vi "SwerveDrive.vi"(0 "x":dbl, 1 "offset":dbl, 2 "Wheel":T1(ring)=enum."FrontLeft", 3 "PWM Counters":cluster{"High":dbl, "Low":dbl}, 5 "y":dbl, 9 "z":dbl, 11 "theta (radians)":dbl, 12 "Enabled":bool=TRUE) -> (4 "twist motor power":dbl, 6 "drive motor power":dbl, 10 "aligned":bool, 13 "angle (radians)":dbl, 14 "Angle Error":dbl, 15 "reversed?":bool)   [LabVIEW 2013]
uses:
  <vilib>/addons/control/pid/pid.llb/PID Advanced (DBL).vi
  <vilib>/addons/control/pid/NI_PID_pid.lvlib
panel:
  in  "PID gains":T2={"proportional gain (Kc)"=0.3, "integral time (Ti, min)"=0.01, "derivative time (Td, min)"=0.0} {"derivative time (Td, min)" format="%.3f"; "integral time (Ti, min)" format="%.3f"; "proportional gain (Kc)" format="%.3f"}
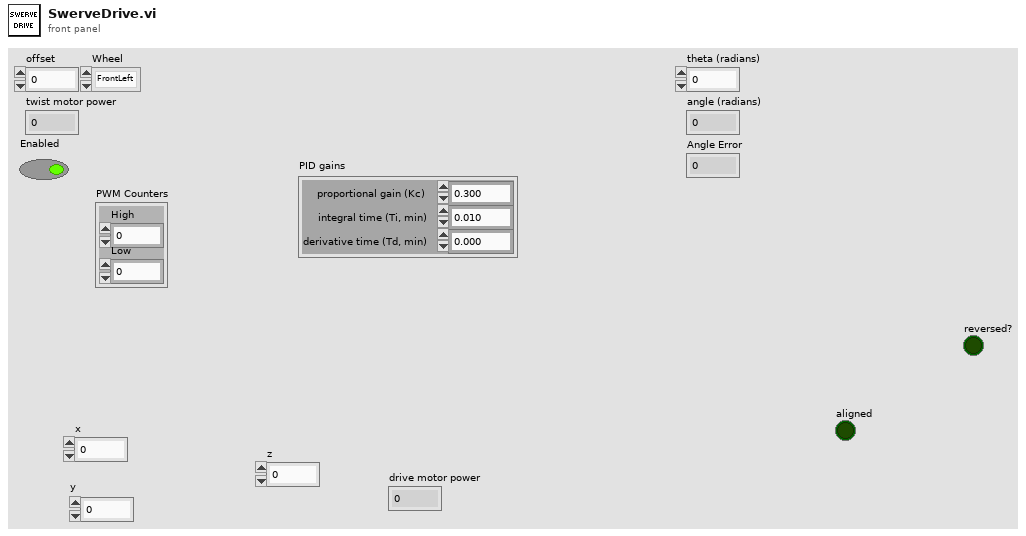
[diagram p1: front panel]
types:
  T1 = enum16{"FrontRight", "FrontLeft", "RearRight", "RearLeft"}
  T2 = cluster{"proportional gain (Kc)":dbl, "integral time (Ti, min)":dbl, "derivative time (Td, min)":dbl}
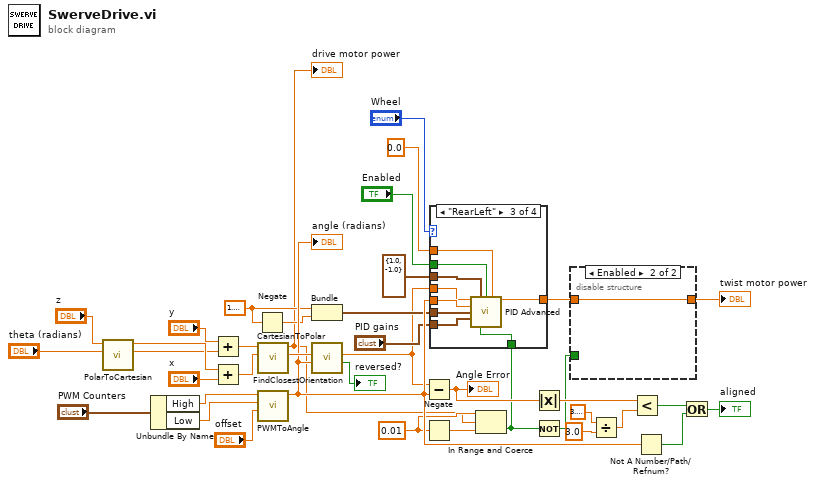
[diagram p0: block diagram]
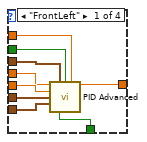
[diagram p2: hidden frame]
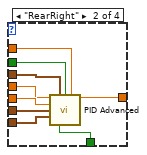
[diagram p3: hidden frame]
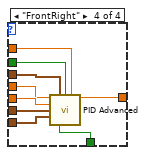
[diagram p4: hidden frame]
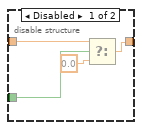
[diagram p5: hidden frame]
diagram:
  w6 = 0.01 ("x")
  w14 = 1.5707963267948966
  n1 = call "PolarToCartesian.vi"("theta (radians)"="theta (radians)", "r"="z") -> ("y"=w35:dbl, "x"=w37:dbl)  [unwired: 8 in]
  n2 = Unbundle By Name("PWM Counters") -> ("High"=w20:dbl, "Low"=w19:dbl)
  n3 = Add(x="y", y=w35) -> (x+y=w29:dbl)
  n4 = Add(x=w37, y="x") -> (x+y=w28:dbl)
  n5 = Negate(x=w14) -> (-x=w13:dbl)
  n6 = call "CartesianToPolar.vi"("y"=w28, "x"=w29) -> ("theta (radians)"=w25:dbl, "r"=w5:dbl)  [unwired: 8 in]
  "drive motor power" <- w5
  n7 = call "PWMToAngle.vi"("official"="offset", "low"=w19, "high"=w20) -> ("angle (radians)"=w16:dbl)  [unwired: 8 in]
  "angle (radians)" <- w16
  n8 = Bundle(w14, w13) -> (w15:cluster{dbl, dbl})  [unwired: 1 in]
  n9 = call "FindClosestOrientation.vi"("current angle (radians)"=w16, "desired angle (radians)"=w25) -> ("reversed?"=→"reversed?":bool, "closest angle (radians)"=w3:dbl)  [unwired: 8 in]
  n10 = Subtract(x=w3, y=w16) -> (x-y=w30:dbl)
  "Angle Error" <- w30
  n11 = Negate(x=w6) -> (-x=w7:dbl)
  n12 = In Range and Coerce(upper limit=w6, x=w5, lower limit=w7) -> (In Range?=w1:bool)  [unwired: 1 out]
  n13 = case shown="\"RearLeft\"" "Wheel" {
    tunnel: w16 -> [w48 w57 w66 w75]
    tunnel: w15 -> [w47 w56 w65 w74]
    tunnel: cluster{"output high":dbl, "output low":dbl} {"output high"=1.0, "output low"=-1.0} ("output range") -> [w46 w55 w64 w73]
    tunnel: "PID gains" -> [w45 w54 w63 w72]
    tunnel: "Enabled" -> [w44 w53 w62 w71]
    tunnel: 0.0 ("manual control") -> [w43 w52 w61 w70]
    tunnel: [w42 w51 w60 w69] -> w8
    tunnel: w3 -> [w41 w50 w59 w68]
    tunnel: w1 -> [w40 w49 w58 w67]
    frame "FrontLeft" {
      n14 = call-poly <vilib>:"PID Advanced.vi"("setpoint"=w41, "output range"=w46, "auto? (T)"=w44, "manual control"=w43, "process variable"=w48, "setpoint range"=w47, "PID gains"=w45, "reinitialize? (F)"=w40) -> ("output"=w42:dbl)  [unwired: 6 in, 1 out]
    }
    frame "RearRight" {
      n15 = call-poly <vilib>:"PID Advanced.vi"("setpoint"=w50, "output range"=w55, "auto? (T)"=w53, "manual control"=w52, "process variable"=w57, "setpoint range"=w56, "PID gains"=w54, "reinitialize? (F)"=w49) -> ("output"=w51:dbl)  [unwired: 6 in, 1 out]
    }
    frame "RearLeft" {
      n16 = call-poly <vilib>:"PID Advanced.vi"("setpoint"=w59, "output range"=w64, "auto? (T)"=w62, "manual control"=w61, "process variable"=w66, "setpoint range"=w65, "PID gains"=w63, "reinitialize? (F)"=w58) -> ("output"=w60:dbl)  [unwired: 6 in, 1 out]
    }
    frame "FrontRight" {
      n17 = call-poly <vilib>:"PID Advanced.vi"("setpoint"=w68, "output range"=w73, "auto? (T)"=w71, "manual control"=w70, "process variable"=w75, "setpoint range"=w74, "PID gains"=w72, "reinitialize? (F)"=w67) -> ("output"=w69:dbl)  [unwired: 6 in, 1 out]
    }
  }
  n18 = Absolute Value(x=w30) -> (abs(x)=w26:dbl)
  n19 = Not(x=w1) -> (.not. x?=w4:bool)
  n20 = disable-structure shown="Enabled" {
    disable-tunnel: [w78 w80] -> w17
    disable-tunnel: w8 -> [w77 w80]
    disable-tunnel: w4 -> [w76 _]
    frame Disabled {
      n21 = Select(t=w77, s=w76, f=0.0) -> (s? t:f=w78:dbl)
    }
    frame Enabled {
    }
  }
  "twist motor power" <- w17
  n22 = Divide(x=3.141592653589793, y=3.0) -> (x/y=w31:dbl)
  n23 = Less?(x=w26, y=w31) -> (x < y?=w27:bool)
  n24 = Not A Number/Path/Refnum?(number/path/refnum=w16) -> (NaN/Path/Refnum?=w23:bool)
  n25 = Or(x=w27, y=w23) -> (x .or. y?=→"aligned":bool)
